vi "CF_Z_Bridge to PGSQL.vi"(8 "error in (no error)":errorcluster, 9 "calibration string":string, 10 "description string":string, 11 "dbl":dbl[](array[numeric])) -> (0 "error out":errorcluster)   [LabVIEW 2013]
uses:
  postgreSQL-lv/Data.PG/Data.PGSQL.lvclass
panel:
  # "CF Impedence Bridge to PGSQL"
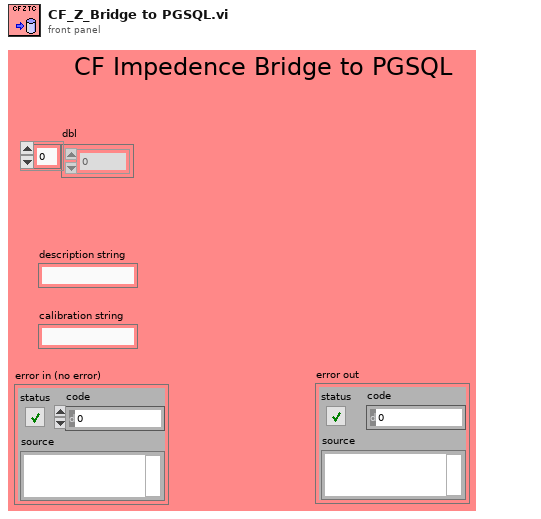
[diagram p1: front panel]
types:
  T1 = cluster{"dbl":dbl[], "description string":string, "calibration string":string}
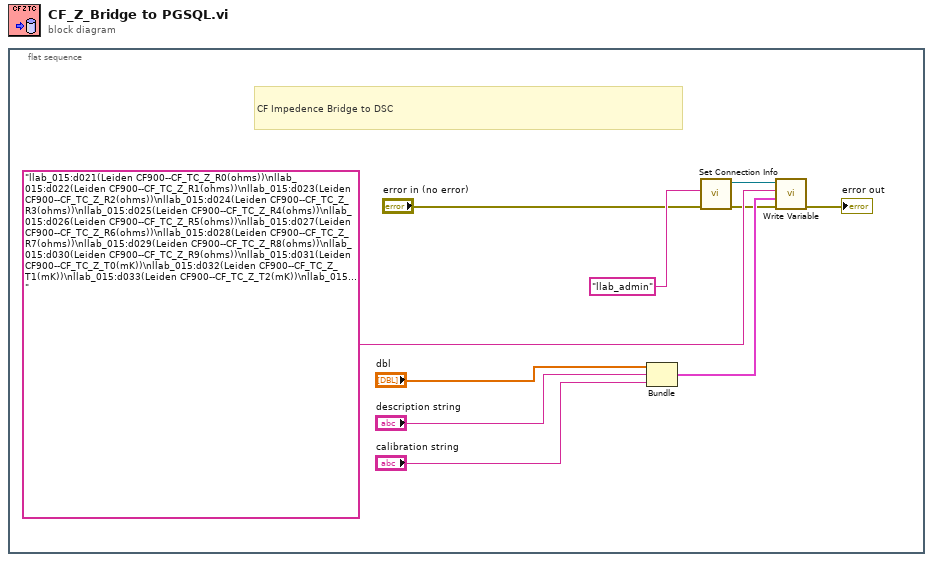
[diagram p0: block diagram]
diagram:
  n1 = flat-sequence {
    frame #0 {
      # "CF Impedence Bridge to DSC"
      n2 = Bundle("dbl"="dbl", "description string"="description string", "calibration string"="calibration string") -> (w6:T1)  [unwired: 1 in]
      n3 = call "Set Connection Info.vi"("username"="llab_admin", "error in (no error)"="error in (no error)") -> ("Data.PG out"=w5:refnum<class "Data.PGSQL.lvclass">, "error out"=w3:errorcluster)  [unwired: 7 in]
      n4 = call "Write Variable.vi"("error in (no error)"=w3, "Data"=w6, "variable"="llab_015:d021(Leiden CF900--CF_TC_Z_R0(ohms))\nllab_015:d022(Leiden CF900--CF_TC_Z_R1(ohms))\nllab_015:d023(Leiden CF900--CF_TC_Z_R2(ohms))\nllab_015:d024(Leiden CF900--CF_TC_Z_R3(ohms))\nllab_015:d025(Leiden CF900--CF_TC_Z_R4(ohms))\nllab_015:d026(Leiden CF900--CF_TC_Z_R5(ohms))\nllab_015:d027(Leiden CF900--CF_TC_Z_R6(ohms))\nllab_015:d028(Leiden CF900--CF_TC_Z_R7(ohms))\nllab_015:d029(Leiden CF900--CF_TC_Z_R8(ohms))\nllab_015:d030(Leiden CF900--CF_TC_Z_R9(ohms))\nllab_015:d031(Leiden CF900--CF_TC_Z_T0(mK))\nllab_015:d032(Leiden CF900--CF_TC_Z_T1(mK))\nllab_015:d033(Leiden CF900--CF_TC_Z_T2(mK))\nllab_015:d034(Leiden CF900--CF_TC_Z_T3(mK))\nllab_015:d035(Leiden CF900--CF_TC_Z_T4(mK))\nllab_015:d036(Leiden CF900--CF_TC_Z_T5(mK))\nllab_015:d037(Leiden CF900--CF_TC_Z_T6(mK))\nllab_015:d038(Leiden CF900--CF_TC_Z_T7(mK))\nllab_015:d039(Leiden CF900--CF_TC_Z_T8(mK))\nllab_015:d040(Leiden CF900--CF_TC_Z_T9(mK))\nllab_015:v002(Leiden CF900--CF_TC_Z_description())\nllab_015:v003(Leiden CF900--CF_TC_Z_calibration())", "Data.PG in"=w5) -> ("error out"=→"error out":errorcluster)  [unwired: 5 in, 2 out]
    }
  }
